vi "Exp12.vi"() -> ()   [LabVIEW 2010]
uses:
  <vilib>/Simulation/Scripting/Companion Diagram/SimConfigNode/SimDog.xnode
  <vilib>/Simulation/Scripting/Companion Diagram/SimConfigNode/SimParams.ctl
  <vilib>/Simulation/Scripting/Companion Diagram/SimConfigNode/_simSolvers.ctl
  <vilib>/Simulation/Implementation/Shared/SIMSCR Execution Mode.ctl
  <vilib>/Platform/TimedLoop/XDataNode/XDataNode.xnode
  <vilib>/Platform/TimedLoop/XDataNode/timing_clust.ctl
  <vilib>/Platform/TimedLoop/XDataNode/nitl_modes.ctl
  <vilib>/Platform/TimedLoop/XDataNode/wakeup.ctl
  <vilib>/Simulation/Implementation/XNodeFramework/SimXNode/SimX.xnode
  <vilib>/Simulation/Implementation/Shared/NILVSim_FinishedLate.vi
  <vilib>/Simulation/DataSources/Implementation/NILVSim Signal Generator.llb/SIM Signal Generator (scalar).vi
  <vilib>/simulation/utility/implementation/sim halt.vi
  <vilib>/Simulation/Implementation/Shared/NILVSim_Manager.vi
  <vilib>/Simulation/Implementation/Shared/NILVSim_FinalizeModel.vi
  <vilib>/Simulation/Implementation/Shared/NILVSim_GetModelError.vi
  <vilib>/Simulation/Implementation/Shared/NILVSim_GetSimErrorInfo.vi
  <vilib>/Simulation/Implementation/Shared/NILVSim_GenerateString.vi
  <vilib>/Simulation/Implementation/Shared/NILVSim_GetBlockNameAndCallChain.vi
  <vilib>/Simulation/Implementation/Shared/NILVSim_GetSimErrorString.vi
  <vilib>/Simulation/Implementation/Shared/NILVSim_GetBlockNameAndCallChainSizes.vi
  <vilib>/Simulation/Implementation/Shared/NILVSim_GetBlockNameAndCallChain Core.vi
  <vilib>/Simulation/Implementation/Shared/SIM Unbundle Sim Info.vi
  <vilib>/Simulation/Implementation/Shared/SIM Bundle Sim Info.vi
  <vilib>/Simulation/Implementation/Shared/NILVSim_Initialize.vi
  <vilib>/dlg_ctls.llb/Space Constant.vi
  Instance           6 13Saved   Exp13 .vi
  Instance          10 13Saved   Exp13 .vi
  Instance           7 13Saved   Exp13 .vi
  Instance          11 13Saved   Exp13 .vi
  Instance           9 13Saved   Exp13 .vi
  Instance          12 13Saved   Exp13 .vi
  Instance           1 13Saved   Exp13 .vi
  Instance           3 13Saved   Exp13 .vi
  Instance           8 13Saved   Exp13 .vi
  <vilib>/Platform/TimedLoop/XDataNode/XDNodeRunTimeDep.lvlib
  <vilib>/Simulation/Implementation/Shared/NI_SIM_Implementation.lvlib
panel:
  out "Figura de Lissajous":cluster{"Y":dbl[], "Y":dbl[]}[](graph)
  in  "OK Button":bool
  in  "Configuração\ndo sinal\nde teste":cluster{"Frequência (rad/s)":dbl}={"Frequência (rad/s)"=2.5}
  out "Medidas":dbl[][](graph)
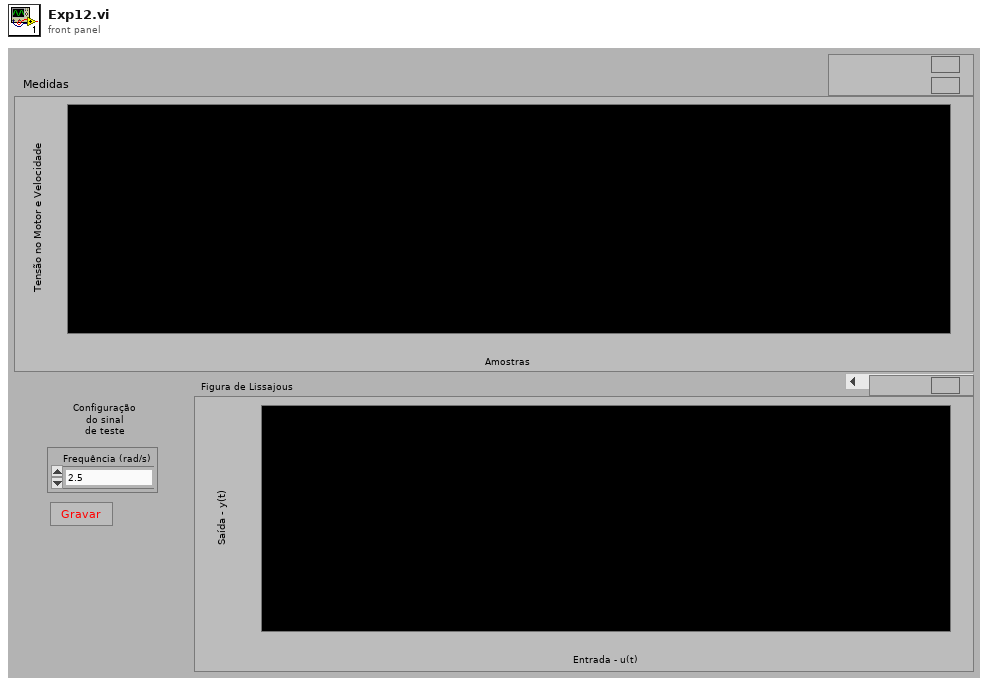
[diagram p1: front panel]
types:
  T1 = typedef "XDNodeRunTimeDep.lvlib/timing_clust.ctl" = cluster{"Expected End [f-1]":u64, "Actual End [f-1]":u64, "Finished Late? [f-1]":bool, "Expected End [i-1]":u64, "Actual End [i-1]":u64, "Finished Late? [i-1]":bool, "Expected Start [i]":u64, "Actual Start [i]":u64, "Expected Start [f]":u64, "Actual Start [f]":u64, "Source Name":string, "Structure Name":string, "Period":i64, "Deadline":i64, "Offset":i64, "Start":i64, "Priority":i32, "Timeout":i32, "Mode":T2, "Wakeup Reason":T3, "Error":errorcluster, "Source Type":string, "Secondary Source Type":string, "Global End Time":u64, "Global Start Time":u64, "Frame Duration":u64, "Iteration Duration":u64, "Assigned CPU":i32, "I/O Scan Engine Mode":u32}
  T2 = typedef "XDNodeRunTimeDep.lvlib/nitl_modes.ctl" = enum32{"No Change", "Process missed periods, maintain original phase", "Discard missed periods, maintain original phase", "Process missed periods, ignore original phase", "Discard missed periods, ignore original phase"}
  T3 = typedef "XDNodeRunTimeDep.lvlib/wakeup.ctl" = enum32{"Normal", "Aborted", "Asynchronous wakeup", "Timing source error", "Timed loop error", "Timeout"}
  T4 = typedef "SimParams.ctl" = cluster{"Initial Time (s)":dbl, "Final Time (s)":dbl, "Step Size (s)":dbl, "ODE Solver":T5, "Minimum Step Size (s)":dbl, "Maximum Step Size (s)":dbl, "Relative Tolerance":dbl, "Absolute Tolerance":dbl, "Software Timing":bool, "Initial Step Size (s)":dbl, "Automatic Fixed Step Size?":bool, "Automatic Discrete Step Size?":bool, "Discrete Step Size (s)":dbl, "Calculate using Time Step":bool, "Solver Wired?":bool, "Prev.Frm.Expected End":u64, "Prev.Frm.Actual End":u64, "Prev.Frm.Finished Late?":bool, "Prev.Iter.Expected End":u64, "Prev.Iter.Actual End":u64, "Prev.Iter.Finished Late?":bool, "Expected Iteration Start":u64, "Actual Iteration Start":u64, "Expected Frame Start":u64, "Actual Frame Start":u64, "Source Name":string, "Name":string, "Period":i64, "Deadline":i64, "Offset":i64, "Start":i64, "Priority":i32, "Timeout":i32, "Processor":i32, "Mode":enum32{"No Change", "Process missed periods, maintain original phase", "Discard missed periods, maintain original phase", "Process missed periods, ignore original phase", "Discard missed periods, ignore original phase"}, "Wakeup reason":enum32{"Normal", "Aborted", "Asynchronous wakeup", "Timing source error", "Timed loop error", "Timeout"}, "Error":errorcluster, "Source Type":string, "Secondary Source Type":string, "Global End Time":u64, "Global Start Time":u64, "Full Solver Reset":bool, "Execution Mode":T6, "Nan/Inf Check":bool, "Custom Solver Library":string, "Solver Is Variable":bool, "custom solver name":string}
  T5 = typedef "_simSolvers.ctl" = enum16{"Runge-Kutta 1 (Euler)", "Runge-Kutta 2", "Runge-Kutta 3", "Runge-Kutta 4", "Runge-Kutta 23 (variable)", "Runge-Kutta 45 (variable)", "BDF (variable)", "Adams-Moulton (variable)", "Rosenbrock (variable)", "Discrete States Only", "Linearizer", "State Query", "Trim Eval", "Custom Solver"}
  T6 = typedef "SIMSCR Execution Mode.ctl" = u16
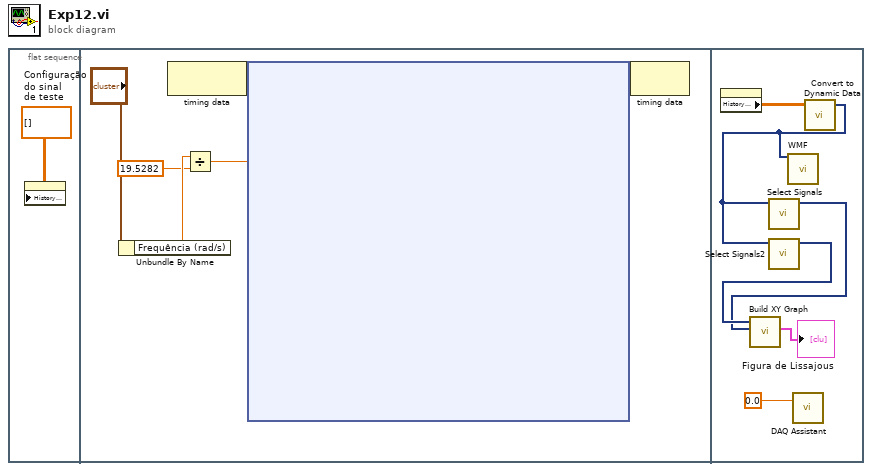
[diagram p0: block diagram]
diagram:
  n1 = flat-sequence {
    frame #0 {
      n2 = property class="WFChart (strict)"("History Data"=dbl[][] []) -> ()  [unwired: 2 in, 2 out]
    }
    frame #1 {
      n3 = Unbundle By Name("Configuração\ndo sinal\nde teste") -> ("Frequência (rad/s)"=w4:dbl)
      n4 = node-c288() -> (w7:variant)  [unwired: 1 in]
      n5 = Divide(x=w4, y=19.5282 ("x")) -> (x/y=w2:dbl)
      n6 = node-c254 ("Control & Simulation Loop")(w7, w2) -> (w6:variant)
      n7 = node-c288(w6) -> ()  [unwired: 1 out]
    }
    frame #2 {
      n8 = property class="WFChart (strict)"() -> ("History Data"=w141:dbl[][])  [unwired: 2 in, 2 out]
      n9 = call "DAQ Assistant"("data"=0.0) -> ()  [unwired: 17 in, 2 out]
      n10 = call "Convert to Dynamic Data"("2D Array"=w141) -> ("Dynamic Data Type"=w139:dynamicdata)  [unwired: 3 in]
      n11 = call "Select Signals"("Signals"=w139) -> ("Signal Out"=w136:dynamicdata)  [unwired: 9 in, 1 out]
      n12 = call "Select Signals2"("Signals"=w139) -> ("Signal Out"=w137:dynamicdata)  [unwired: 9 in, 1 out]
      n13 = call "Build XY Graph"("Y Input"=w136, "X Input"=w137) -> ("XY Graph"=→"Figura de Lissajous":cluster{"Y":dbl[], "Y":dbl[]}[])  [unwired: 8 in, 1 out]
      n14 = call "WMF"("Signals"=w139) -> ()  [unwired: 16 in, 3 out]
    }
  }
